vi "Write Packages.vi"(8 "error in (no error)":errorcluster, 10 "Packages":refnum<class "Package.lvclass">[](array[class]), 11 "Repo in":refnum<class "Repo.lvclass">) -> (0 "error out":errorcluster, 3 "Repo out":refnum<class "Repo.lvclass">)   [LabVIEW 2020, in "Packages.lvlib" / "Repo.lvclass"]
uses:
  Repo.lvclass
  Package_class/Package.lvclass
  Repo.lvclass/Repo.ctl
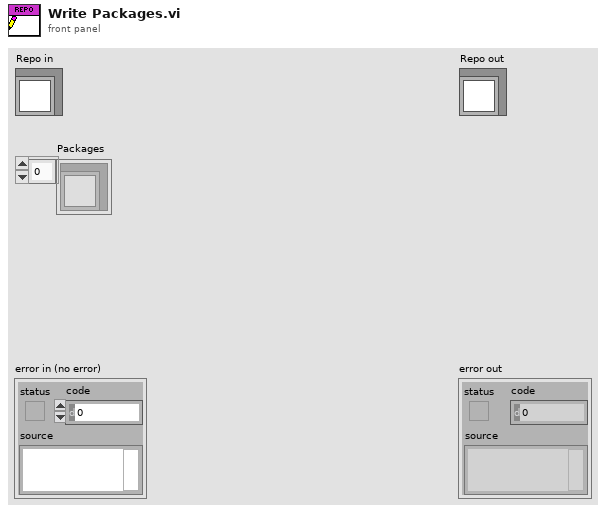
[diagram p1: front panel]
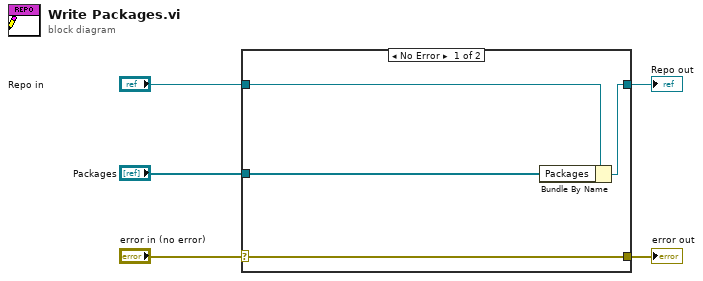
[diagram p0: block diagram]
diagram:
  n1 = case shown="No Error" "error in (no error)" {
    selector: "error in (no error)" -> [w9 w10]
    tunnel: [w9 w10] -> w4
    tunnel: [w7 w11] -> w2
    tunnel: "Repo in" -> [w8 w11]
    tunnel: "Packages" -> [w6 _]
    frame No Error {
      n2 = Bundle By Name(cluster=w8, "Packages"=w6) -> (w7:refnum<class "Repo.lvclass">)
    }
    frame Error {
    }
  }
  "error out" <- w4
  "Repo out" <- w2
